vi "loadScopeTraceFromFile.vi"(8 "error in (no error)":errorcluster, 10 "file path (dialog if empty)":path, 11 "WaveformGraph in":refnum<vi>) -> (0 "error out":errorcluster, 1 "Array 2":waveform(dbl)[](array[waveform]), 2 "number of waveforms":i32, 3 "Array":string[](array[string]))   [LabVIEW 2013]
uses:
  <instrlib>/niHWS/nihws.llb/niHWS Open File Permissions ID.ctl
  <instrlib>/niHWS/nihws.llb/niHWS Set Wfm DBL Attribute ID.ctl
  <instrlib>/niHWS/nihws.llb/niHWS Get Wfm DBL Attribute.vi
  <instrlib>/niHWS/nihws.llb/niHWS Read Analog WDT.vi
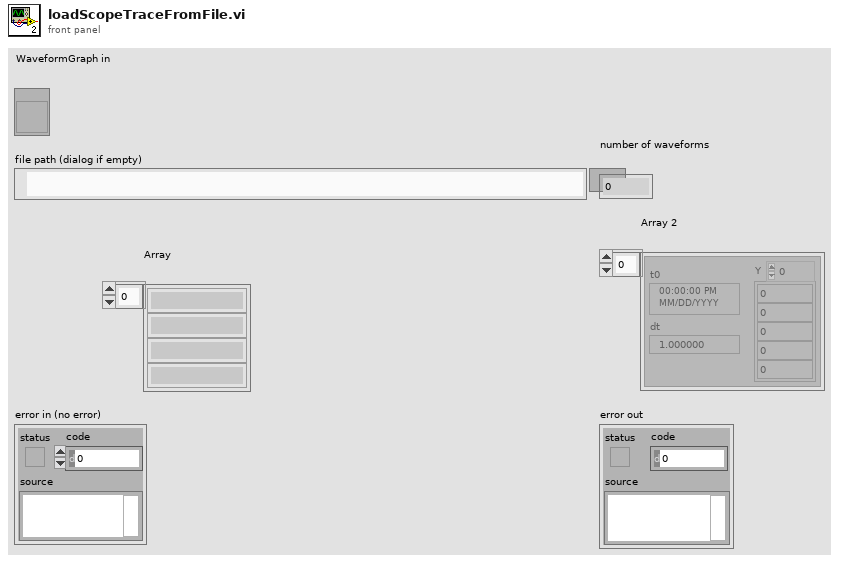
[diagram p1: front panel]
types:
  T1 = typedef "niHWS Open File Permissions ID.ctl" = enum32{"Read Only", "Read/Write Existing", "Read/Write/Create New", "Read/Write/Create New Always"}
  T2 = typedef "niHWS Set Wfm DBL Attribute ID.ctl" = u32
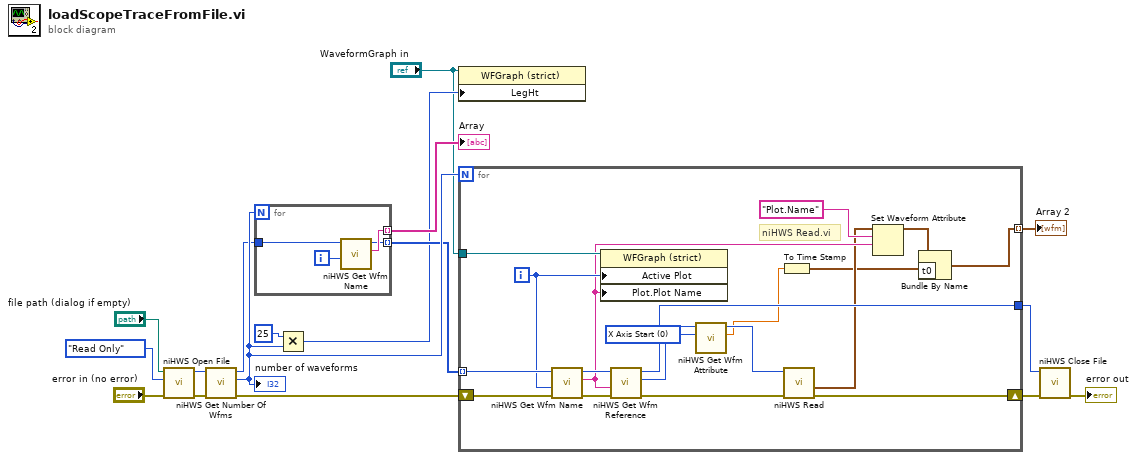
[diagram p0: block diagram]
diagram:
  n1 = call <instrlib>:"niHWS Open File.vi"("error in (no error)"="error in (no error)", "permissions (0:read only)"=niHWS_Open_File_Permissions_ID."Read Only", "file path"="file path (dialog if empty)") -> ("error out"=w5:errorcluster, "file handle"=w6:u32)  [unwired: 7 in]
  n2 = call <instrlib>:"niHWS Get Number Of Wfms.vi"("error in (no error)"=w5, "file handle in"=w6) -> ("error out"=w4:errorcluster, "number of waveforms"=w17:i32, "file handle out"=w14:u32)  [unwired: 7 in]
  "number of waveforms" <- w17
  n3 = for {
    N: w17 -> [_]
    tunnel: w14 -> [w21]
    tunnel: [w20] -> w16 mode=indexing
    tunnel: [w19] -> w15 mode=indexing
    i -> [w18]
    n4 = call <instrlib>:"niHWS Get Wfm Name.vi"("waveform index (0)"=w18, "file handle in"=w21) -> ("waveform name"=w20:string, "file handle out"=w19:u32)  [unwired: 7 in, 1 out]
  }
  "Array" <- w16
  n5 = Multiply(x=u32 25 ("Legend:Size:Height"), y=w17) -> (x*y=w13:u32)
  n6 = property on="Property Node" class="WFGraph (strict)"(reference="WaveformGraph in", "LegHt"=w13) -> ()  [unwired: 1 in, 2 out]
  n7 = for {
    N: w17 -> [_]
    tunnel: [w22] -> w8 mode=indexing
    tunnel: w15 -> [w39] mode=indexing
    tunnel: [w36] -> w11
    shift-right: [w38] -> w10
    shift-left: w4 -> [w40]
    tunnel: "WaveformGraph in" -> [w32]
    i -> [w33]
    w26 = T2 0 items=["X Axis Start"=0, "X Axis Increment"=1, "Y Axis Minimum"=3, "Y Axis Maximum"=4] ("attribute ID")
    # "niHWS Read.vi"
    n8 = call <instrlib>:"niHWS Get Wfm Name.vi"("error in (no error)"=w40, "waveform index (0)"=w33, "file handle in"=w39) -> ("error out"=w35:errorcluster, "waveform name"=w31:string, "file handle out"=w37:u32)  [unwired: 6 in]
    n9 = property on="Property Node" class="WFGraph (strict)"(reference=w32, "Active Plot"=w33, "Plot.Plot Name"=w31) -> ()  [unwired: 1 in, 2 out]
    n10 = call <instrlib>:"niHWS Get Wfm Reference.vi"("error in (no error)"=w35, "waveform name (empty)"=w31, "file handle in"=w37) -> ("error out"=w34:errorcluster, "waveform reference"=w29:u32, "file handle out"=w36:u32)  [unwired: 6 in]
    n11 = call-poly <instrlib>:"niHWS Get Wfm Attribute.vi"("attribute ID"=w26, "waveform reference in"=w29) -> ("attribute value"=w24:dbl, "waveform reference out"=w28:u32)  [unwired: 7 in, 1 out]
    n12 = To Time Stamp(1:w24) -> (0:w23:timestamp)
    n13 = call-poly <instrlib>:"niHWS Read.vi"("error in (no error)"=w34, "waveform reference in"=w28) -> ("error out"=w38:errorcluster, "analog waveform"=w27:waveform(dbl))  [unwired: 6 in, 2 out]
    n14 = Set Waveform Attribute(5:w31, 6:"Plot.Name" ("name"), 7:w27) -> (3:w25:waveform(dbl))  [unwired: 1 in, 2 out]
    n15 = Bundle By Name(cluster=w25, "t0"=w23) -> (w22:waveform(dbl))
  }
  "Array 2" <- w8
  n16 = call <instrlib>:"niHWS Close File.vi"("error in (no error)"=w10, "file handle"=w11) -> ("error out"=→"error out":errorcluster)  [unwired: 9 in]
